vi "Elevator Loop.vi"   [LabVIEW 2014]
uses:
  Common Code/Elevator Status.ctl
  Common Code/Elevator Mode.ctl
  Common Code/Auto Elevator Indicators.ctl
  Common Code/Elevator State.ctl
  Common Code/Change Detect Int.vi
  Robot Global Data.vi
  <vilib>/Rock Robotics/WPI/Solenoid/Deprecated/WPI_SolenoidSetBool.vi
types:
  T1 = typedef "Elevator Status.ctl" = cluster{"Height":dbl, "Enc Value":dbl, "Limit Override":bool, "Mode":T2, "High IR":bool, "Motor Out":dbl, "Ping Detect":bool, "Auto Elevator Indicators":T3, "Master Current":dbl, "Slave Current":dbl, "High Current":bool, "Current Tripped":bool, "Top Limit":bool, "Bottom Limit":bool, "Eject Piston":bool, "Stabilizer":bool, "Finger":bool, "Finger Height":dbl, "Finger Raw":dbl, "Finger at Bottom":bool}
  T2 = typedef "Elevator Mode.ctl" = enum16{"Manual", "Safe", "Auto"}
  T3 = typedef "Auto Elevator Indicators.ctl" = cluster{"Target Out":dbl, "Storing Trashcan?":bool, "State":T4, "In Range":bool, "Store Can Command":bool, "HP Load":bool}
  T4 = typedef "Elevator State.ctl" = enum16{"Idle", "Goto Load Position", "Wait for Load", "Load Drop", "Load Lift", "Drop Stack", "Goto Eject Position", "Eject ", "Raise Trashcan", "Open Stabilizer", "Untip Drop", "Untip Wait", "Untip Lift", "Abort Load", "HP Load Wait", "HP Load Drop", "HP Load Lift", "HP Load Abort", "Close Stabilizer", "HP Load Unfinish", "HP Load Score", "HP Load Finish", "HP Goto Finish Down", "HP Goto Finish Up", "Full"}
  T5 = typedef "Elevator Control Command.ctl" = cluster{"Command":T6, "Manual Motor Out":dbl, "Manual Eject Piston":bool, "Mode":T2, "Override Limits":bool, "Manual Stabilizer":bool, "Manual Finger":bool, "Store Trashcan?":bool, "Hold Low?":bool, "Idle Mode":T7, "HP Load":bool, "Unstick":bool, "Raw Height Set":dbl, "Force Store":bool}
  T6 = typedef "Elevator Command.ctl" = enum16{"Idle", "Load 1", "Load 2", "Load 3", "Drop Stack", "Eject Stack", "Untip Trashcan", "Load Trashcan", "HP Load", "HP Score"}
  T7 = typedef "Elevator Idle Mode.ctl" = enum16{"Load 1", "Load 2", "Load 3", "Load Can", "Untip Can", "Step Load", "Drop Stack", "Raw Height"}
  T8 = typedef "WPI_DigitalInputDevRef.ctl" = cluster{"DevStatus":errorcluster, "DIO Channel":T9, "Controller":T10}
  T9 = typedef "FPGA_DIOChannel.ctl" = enum8{"DIO 0", "DIO 1", "DIO 2", "DIO 3", "DIO 4", "DIO 5", "DIO 6", "DIO 7", "DIO 8", "DIO 9", "DIO MXP 0", "DIO MXP 1", "DIO MXP 2", "DIO MXP 3", "DIO MXP 4", "DIO MXP 5", "DIO MXP 6", "DIO MXP 7", "DIO MXP 8", "DIO MXP 9", "DIO MXP 10", "DIO MXP 11", "DIO MXP 12", "DIO MXP 13", "DIO MXP 14", "DIO MXP 15", "Invalid"}
  T10 = typedef "FPGA_TypedefDigitalModule.ctl" = enum16{"Controller 1"}
  T11 = typedef "WPI_MotorControlDeviceRef.ctl" = cluster{"DeviceStatus":errorcluster, "Type":T12, "PWM":cluster{"Controller":T10, "PWM Channel":T13, "DeadBand":T14}, "CAN":cluster{"Device Number":u8, "Control Mode":T15, "Semaphore":T16, "Max Vout":dbl, "TalonSRX Control Mode":T17}, "Invert":bool, "TransformRef":T18, "InvTransformRef":T18}
  T12 = typedef "WPI_MotorControlType.ctl" = enum16{"PWM", "CAN", "CANTalonSRX"}
  T13 = typedef "FPGA_DIOPWMChannel.ctl" = enum8{"PWM 0", "PWM 1", "PWM 2", "PWM 3", "PWM 4", "PWM 5", "PWM 6", "PWM 7", "PWM 8", "PWM 9", "PWM MXP 0", "PWM MXP 1", "PWM MXP 2", "PWM MXP 3", "PWM MXP 4", "PWM MXP 5", "PWM MXP 6", "PWM MXP 7", "PWM MXP 8", "PWM MXP 9", "Invalid"}
  T14 = typedef "WPI_PWMDeadband.ctl" = cluster{"Name":string, "maxPositivePwm":i32, "minPositivePwm":i32, "centerPwm":i32, "maxNegativePwm":i32, "minNegativePwm":i32, "angularRange":u16}
  T15 = typedef "WPI_CANJaguar_ControlMode.ctl" = enum8{"Percent VBus", "Current", "Speed", "Position", "Voltage"}
  T16 = typedef "Semaphore RefNum" = refnum<k1>
  T17 = typedef "WPI_CANTalonSRX_APIControlMode.ctl" = enum8{"Percent VBus", "Speed", "Position", "Slave", "Unchanged / Invalid"}
  T18 = typedef "WPI_PWMTransform_ConPane.ctl" = refnum<vi>
  T19 = typedef "WPI_SolenoidDevRef.ctl" = cluster{"DevStatus":errorcluster, "Pneumatics Control Module":u8, "Forward Solenoid Channel":T20, "Reverse Solenoid Channel":T20}
  T20 = typedef "WPI_SolenoidChannel.ctl" = enum8{"Solenoid 0", "Solenoid 1", "Solenoid 2", "Solenoid 3", "Solenoid 4", "Solenoid 5", "Solenoid 6", "Solenoid 7", "Invalid"}
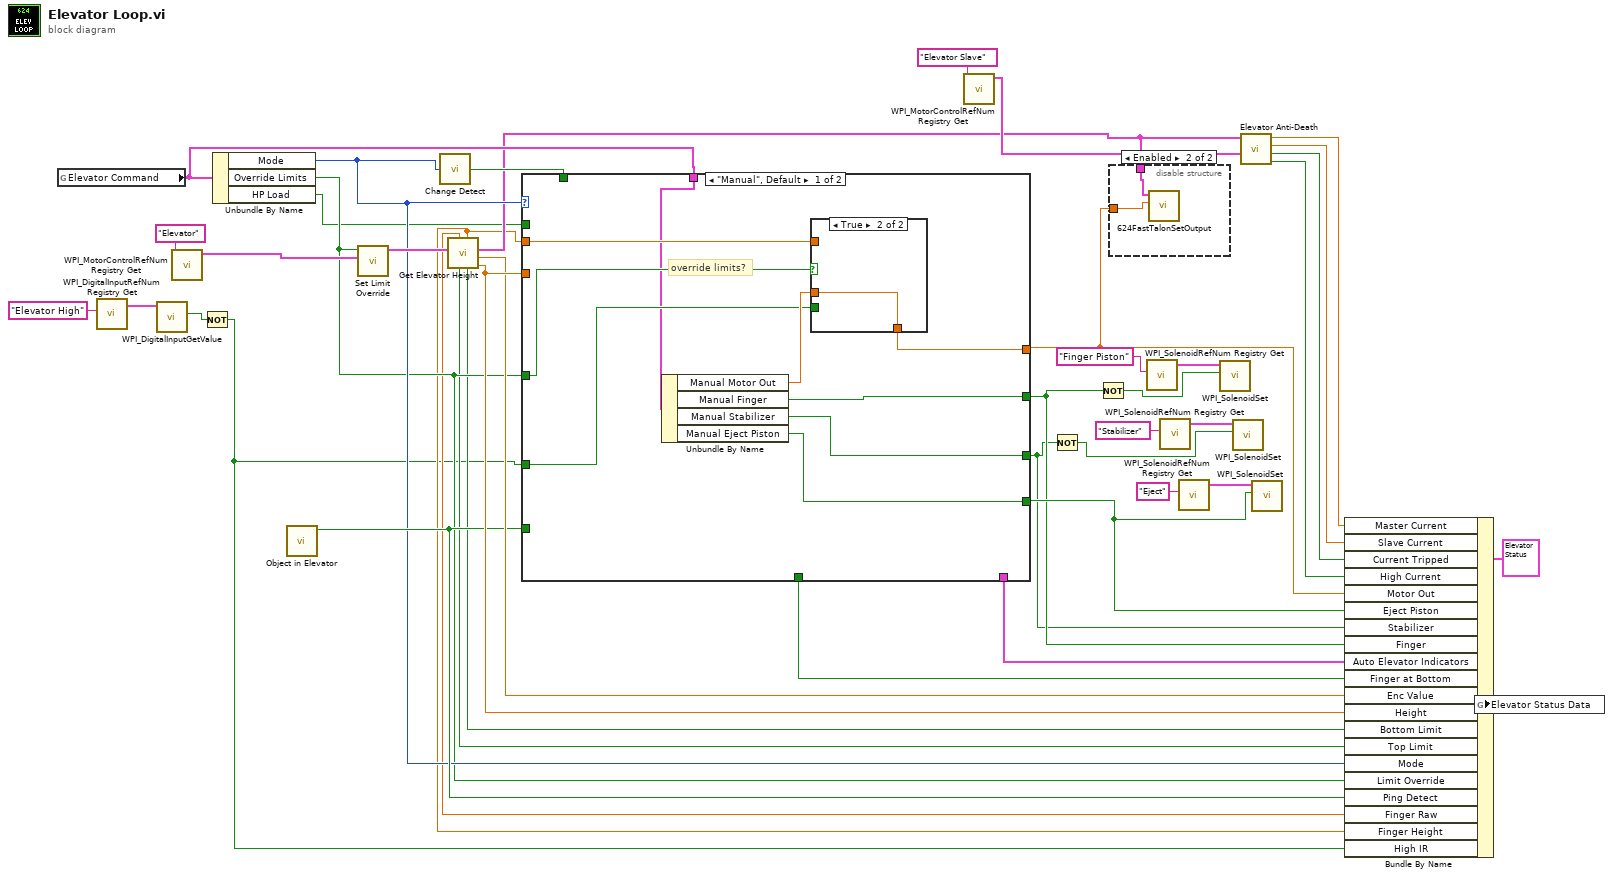
[diagram p0: block diagram]
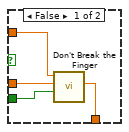
[diagram p2: hidden frame]
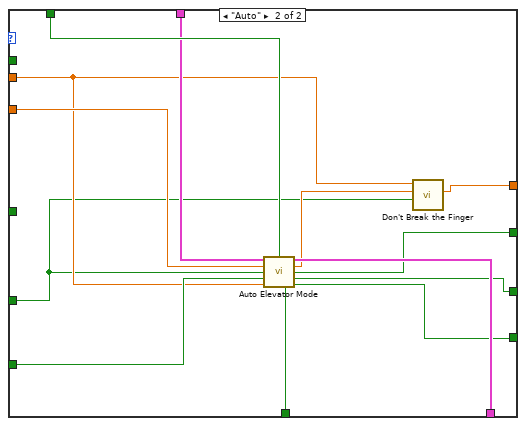
[diagram p3: hidden frame]
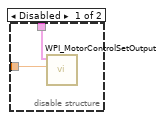
[diagram p4: hidden frame]
diagram:
  n1 = global read "Robot Global Data.vi" "Elevator Command"() -> (w23:T5)
  n2 = call <vilib>:"WPI_DigitalInputRefNum Registry Get.vi"("refnum name"="Elevator High") -> ("DigitalInputDevRef"=w3:T8)  [unwired: 9 in, 1 out]
  n3 = call <vilib>:"WPI_DigitalInputGetValue.vi"("DigitalInputDevRef"=w3) -> ("Value"=w2:bool)  [unwired: 8 in, 2 out]
  n4 = call <vilib>:"WPI_MotorControlRefNum Registry Get.vi"("refnum name"="Elevator") -> ("MotorControlDevRef"=w39:T11)  [unwired: 9 in, 1 out]
  n5 = Not(x=w2) -> (.not. x?=w1:bool)
  n6 = Unbundle By Name(w23) -> ("Mode"=w26:T2, "Override Limits"=w24:bool, "HP Load"=w10:bool)
  n7 = call "Object in Elevator.vi"() -> ("Ping Detect"=w27:bool)  [unwired: 11 in]
  n8 = call "Set Limit Override.vi"("MotorControlDevRef"=w39, "Override Limits"=w24) -> ("CAN Talon SRX Ref Out"=w38:T11)  [unwired: 9 in]
  n9 = call-poly "Change Detect.vi"("In"=w26) -> ("Changed?"=w30:bool)
  n10 = call "Get Elevator Height.vi"("MotorControlDevRef"=w38) -> ("Height"=w33:dbl, "Encoder Value"=w28:dbl, "CAN Talon SRX Ref Out"=w15:T11, "Bottom Limit Switch"=w22:bool, "Finger Height"=w8:dbl, "Top Limit Switch"=w21:bool, "Finger Raw"=w9:dbl)  [unwired: 4 in]
  n11 = case shown="\"Manual\", Default" w26 {
    tunnel: [w47 w61] -> w31
    tunnel: w33 -> [_ w65]
    tunnel: [w51 w67] -> w6
    tunnel: [w50 w68] -> w19
    tunnel: [w49 w62] -> w32
    tunnel: [_ w69] -> w20
    tunnel: w30 -> [_ w66]
    tunnel: w27 -> [_ w63]
    tunnel: w24 -> [w44 _]
    tunnel: w23 -> [w43 w64]
    tunnel: w10 -> [_ _]
    tunnel: w8 -> [w46 w59]
    tunnel: [_ w58] -> w7
    tunnel: w1 -> [w45 w57]
    frame "Manual", Default {
      # "override limits?"
      n12 = Unbundle By Name(w43) -> ("Manual Motor Out"=w48:dbl, "Manual Finger"=w50:bool, "Manual Stabilizer"=w51:bool, "Manual Eject Piston"=w49:bool)
      n13 = case shown="True" w44 {
        tunnel: w48 -> [w55 w56]
        tunnel: [w54 w56] -> w47
        tunnel: w46 -> [w53 _]
        tunnel: w45 -> [w52 _]
        frame False {
          n14 = call "Don't Break the Finger.vi"("High IR"=w52, "Elevator motor in"=w55, "Finger Height"=w53) -> ("Elevator motor out"=w54:dbl)  [unwired: 8 in]
        }
        frame True {
        }
      }
    }
    frame "Auto" {
      n15 = call "Auto Elevator Mode.vi"("Elevator Command"=w64, "reinitialize? (F)"=w66, "Current Position"=w65, "High IR"=w57, "Object In?"=w63, "Finger Height"=w59) -> ("Auto Elevator Indicators"=w69:T3, "output"=w60:dbl, "Finger Out"=w68:bool, "Stabilizer Out"=w67:bool, "Finger at bottom"=w58:bool, "Eject Out"=w62:bool)  [unwired: 4 in]
      n16 = call "Don't Break the Finger.vi"("High IR"=w57, "Elevator motor in"=w60, "Finger Height"=w59) -> ("Elevator motor out"=w61:dbl)  [unwired: 8 in]
    }
  }
  n17 = call <vilib>:"WPI_MotorControlRefNum Registry Get.vi"("refnum name"="Elevator Slave") -> ("MotorControlDevRef"=w16:T11)  [unwired: 9 in, 1 out]
  n18 = Not(x=w6) -> (.not. x?=w5:bool)
  n19 = Not(x=w19) -> (.not. x?=w18:bool)
  n20 = disable-structure shown="Enabled" {
    disable-tunnel: w15 -> [w71 w73]
    disable-tunnel: w31 -> [w70 w72]
    frame Disabled {
      n21 = call <vilib>:"WPI_MotorControlSetOutput.vi"("Output"=w70, "MotorControlDevRef"=w71) -> ()  [unwired: 7 in, 3 out]
    }
    frame Enabled {
      n22 = call "624FastTalonSetOutput.vi"("Output"=w72, "MotorControlDevRef"=w73) -> ()  [unwired: 8 in, 2 out]
    }
  }
  n23 = call <vilib>:"WPI_SolenoidRefNum Registry Get.vi"("refnum name"="Finger Piston") -> ("SolenoidDevRef"=w35:T19)  [unwired: 9 in, 1 out]
  n24 = call <vilib>:"WPI_SolenoidRefNum Registry Get.vi"("refnum name"="Stabilizer") -> ("SolenoidDevRef"=w37:T19)  [unwired: 9 in, 1 out]
  n25 = call <vilib>:"WPI_SolenoidRefNum Registry Get.vi"("refnum name"="Eject") -> ("SolenoidDevRef"=w41:T19)  [unwired: 9 in, 1 out]
  n26 = call-poly <vilib>:"WPI_SolenoidSet.vi"("Value"=w18, "SolenoidDevRef"=w35) -> ()  [unwired: 8 in, 2 out]
  n27 = call-poly <vilib>:"WPI_SolenoidSet.vi"("Value"=w5, "SolenoidDevRef"=w37) -> ()  [unwired: 8 in, 2 out]
  n28 = call "Elevator Anti-Death.vi"("Slave"=w16, "Master"=w15) -> ("High Current"=w11:bool, "Current Tripped"=w12:bool, "Slave Current"=w13:dbl, "Master Current"=w14:dbl)  [unwired: 6 in]
  n29 = call-poly <vilib>:"WPI_SolenoidSet.vi"("Value"=w32, "SolenoidDevRef"=w41) -> ()  [unwired: 8 in, 2 out]
  n30 = Bundle By Name(cluster=T1 {"Height"=0.0, "Enc Value"=0.0, "Limit Override"=FALSE, "Mode"=enum."Manual", "High IR"=FALSE, "Motor Out"=0.0, "Ping Detect"=FALSE, "Auto Elevator Indicators"={"Target Out"=0.0, "Storing Trashcan?"=FALSE, "State"=enum."Idle", "In Range"=FALSE, "Store Can Command"=FALSE, "HP Load"=FALSE}, "Master Current"=0.0, "Slave Current"=0.0, "High Current"=FALSE, "Current Tripped"=FALSE, "Top Limit"=FALSE, "Bottom Limit"=FALSE, "Eject Piston"=FALSE, "Stabilizer"=FALSE, "Finger"=FALSE, "Finger Height"=0.0, "Finger Raw"=0.0, "Finger at Bottom"=FALSE} ("Elevator Status Data"), "Master Current"=w14, "Slave Current"=w13, "Current Tripped"=w12, "High Current"=w11, "Motor Out"=w31, "Eject Piston"=w32, "Stabilizer"=w6, "Finger"=w19, "Auto Elevator Indicators"=w20, "Finger at Bottom"=w7, "Enc Value"=w28, "Height"=w33, "Bottom Limit"=w22, "Top Limit"=w21, "Mode"=w26, "Limit Override"=w24, "Ping Detect"=w27, "Finger Raw"=w9, "Finger Height"=w8, "High IR"=w1) -> (w29:T1)
  n31 = global write "Robot Global Data.vi" "Elevator Status Data"(w29) -> ()
